vi "hydrolyse_reactor_merge.vi"(10 "hydrolysis_path":path) -> ()   [LabVIEW 2019]
uses:
  lib/libSimulationControl/libSimulationControl.lvlib
  lib/libFileFunctions/libFileFunctions.lvlib
panel:
  # "*******************************************************************\nBiogas Plant Control\n\nAuthor: Paul Zügel\nGCSC-Frankfurt am Main 2020\n\n*******************************************************************"
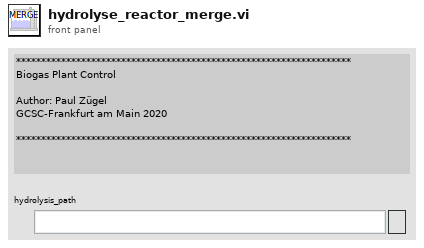
[diagram p1: front panel]
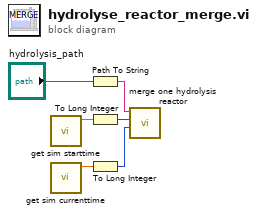
[diagram p0: block diagram]
diagram:
  n1 = call "get sim starttime.vi"() -> ("sim_starttime"=w3:dbl)  [unwired: 10 in, 1 out]
  n2 = call "get sim currenttime.vi"() -> ("current_time"=w4:dbl)  [unwired: 10 in, 1 out]
  n3 = Path To String(path="hydrolysis_path") -> (string=w5:string)
  n4 = To Long Integer(number=w3) -> (32bit integer=w2:i32)
  n5 = To Long Integer(number=w4) -> (32bit integer=w1:i32)
  n6 = call "merge one hydrolysis reactor.vi"("current_starttime"=w1, "simulation_starttime"=w2, "working_dir"=w5) -> ()  [unwired: 8 in, 1 out]
